vi "Quaternion_New_Default.vi"() -> (3 "out Quaternion":T1={"R"=1.0, "V"=[0.0, 0.0, 0.0]})   [LabVIEW 2019, in "Trajectory_Library.lvlib"]
doc: "Constructs a quaternion with a default angle of 0 degrees\n\nParameters:\n -- None -- \n\nReturns:\n - out Quaternion -- Created data cluster"
uses:
  Trajectory_Library.lvlib
  QUATERNION.ctl
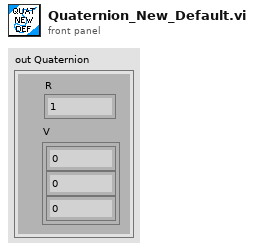
[diagram p1: front panel]
types:
  T1 = typedef "Trajectory_Library.lvlib/QUATERNION.ctl" = cluster{"R":dbl, "V":dbl[]}
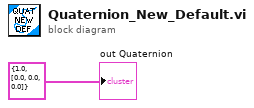
[diagram p0: block diagram]
diagram:
  "out Quaternion" <- T1 {"R"=1.0, "V"=[0.0, 0.0, 0.0]} ("sumPOSE")
